vi "Connect to Error Handles.vi"(8 "error in":errorcluster, 9 "Timeout (ms)":u16, 11 "VS Plugin Inline Async API in":refnum<class "VS Plugin Inline Async API.lvclass">) -> (0 "error out":errorcluster, 3 "VS Plugin Inline Async API out":refnum<class "VS Plugin Inline Async API.lvclass">)   [LabVIEW 2024, in "VS Plugin Inline Async API.lvlib" / "VS Plugin Inline Async API.lvclass"]
uses:
  VS Plugin Inline Async API.lvclass
  VS Plugin Inline Async API.lvclass/VS Plugin Inline Async API.ctl
  <vilib>/ErrorRing/Error Ring.xnode
  VS Plugin Inline Async API.lvlib
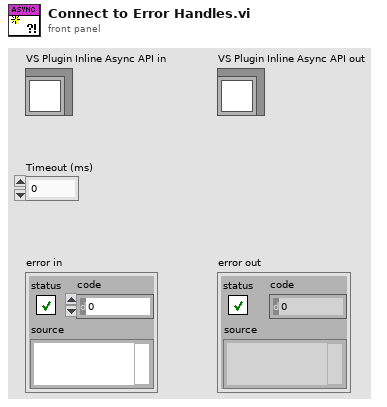
[diagram p1: front panel]
types:
  T1 = cluster{"read mode":enum16{"polling", "blocking"}, "write mode":enum16{"polling", "blocking"}}
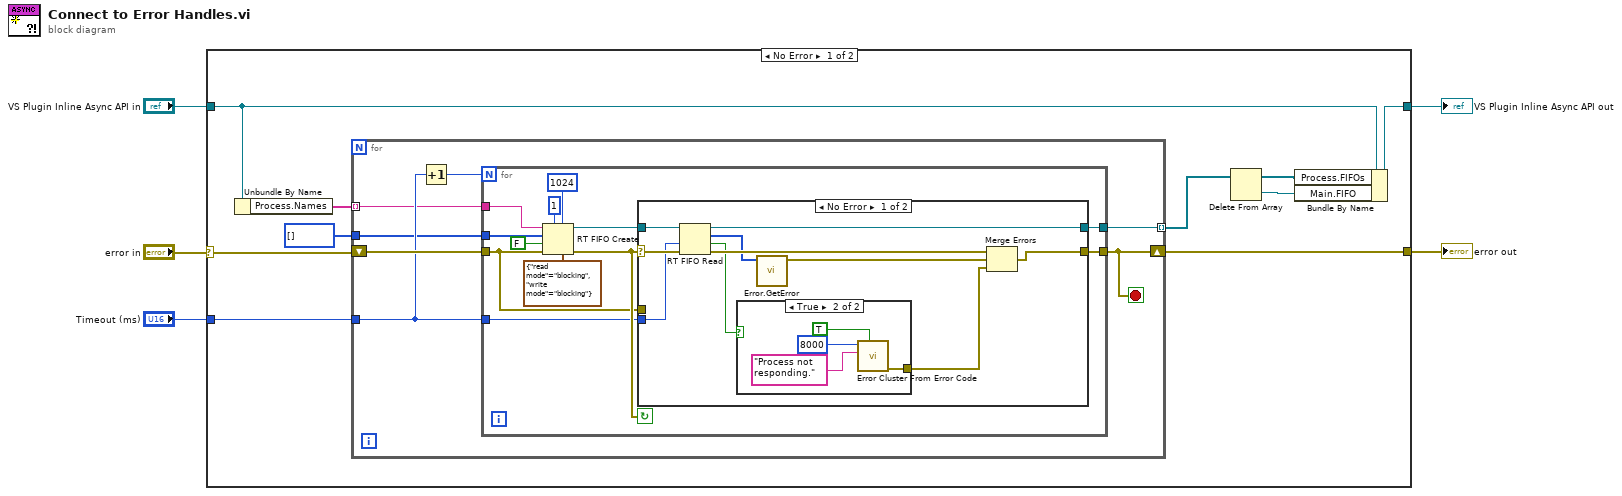
[diagram p0: block diagram]
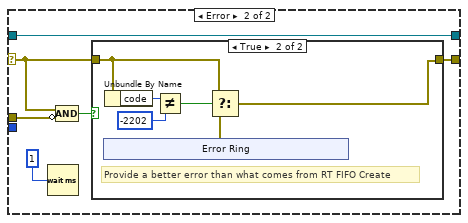
[diagram p3: hidden frame]
diagram:
  n1 = case shown="No Error" "error in" {
    selector: "error in" -> [w15 w67]
    tunnel: [w14 w67] -> w4
    tunnel: "Timeout (ms)" -> [w13 _]
    tunnel: "VS Plugin Inline Async API in" -> [w11 w66]
    tunnel: [w12 w66] -> w1
    frame No Error {
      n2 = Unbundle By Name(w11) -> ("Process.Names"=w10:string[])
      n3 = for {
        shift-right: [w21] -> w14
        shift-left: w15 -> [w22]
        tunnel: [w20] -> w9 mode=indexing
        tunnel: w13 -> [w18]
        tunnel: w10 -> [w17] mode=indexing
        tunnel: u8[] [] -> [w16]
        stop <- w21 stop-if-true
        n4 = Increment(x=w18) -> (x+1=w19:u16)
        n5 = for {
          N: w19 -> [_]
          tunnel: [w30] -> w20
          tunnel: w18 -> [w28]
          tunnel: w22 -> [w32]
          tunnel: [w34] -> w21
          tunnel: w17 -> [w27]
          tunnel: w16 -> [w24]
          stop <- w33 continue-if-true
          n6 = RT FIFO Create(0:w27, 1:w24, 2:FALSE ("create if not found? (T)"), 3:w32, 4:u32 1 ("size (10)"), 6:u32 1024 ("elements in array (1)"), 7:T1 {"read mode"=enum."blocking", "write mode"=enum."blocking"} ("r/w modes (polling,polling)")) -> (8:w29:refnum<k33>, 11:w33:errorcluster)  [unwired: 1 in, 1 out]
          n7 = case shown="No Error" w33 {
            selector: w33 -> [w44 w53]
            tunnel: [w42 w52] -> w34
            tunnel: [w38 w51] -> w30
            tunnel: w29 -> [w39 w51]
            tunnel: w28 -> [w37 _]
            tunnel: w32 -> [_ w54]
            frame No Error {
              n8 = RT FIFO Read(0:w39, 2:w37, 3:w44) -> (8:w38:refnum<k33>, 9:w35:u8[], 10:w36:bool, 11:w43:errorcluster)  [unwired: 1 in, 1 out]
              n9 = case shown="True" w36 {
                tunnel: [_ w48] -> w41
                frame False {
                }
                frame True {
                  n10 = call <vilib>:"Error Cluster From Error Code.vi"("show call chain? (False)"=TRUE, "error message (\"\")"="Process not responding." ("source"), "error code (0)"=8000) -> ("error out"=w48:errorcluster)  [unwired: 6 in]
                }
              }
              n11 = call "Error.GetError.vi"("Msg"=w35) -> ("error out"=w40:errorcluster)  [unwired: 10 in]
              n12 = Merge Errors(w43, w40, w41) -> (w42:errorcluster)
            }
            frame Error {
              n13 = Wait (ms)(milliseconds to wait=u32 1) -> ()  [unwired: 1 out]
              n14 = Compound Arithmetic op=AND(w53, invert w54) -> (w49:bool)
              n15 = case shown="True" w49 {
                tunnel: w53 -> [w55 w61]
                tunnel: [w55 w59] -> w52
                frame False {
                  # "No new error from RT FIFO Create"
                }
                frame True {
                  # "Provide a better error than what comes from RT FIFO Create"
                  n16 = xnode "Error Ring"() -> ("error out"=w60:errorcluster)
                  n17 = Unbundle By Name(w61) -> ("code"=w58:i32)
                  n18 = Not Equal?(x=w58, y=-2202) -> (x != y?=w56:bool)
                  n19 = Select(t=w61, s=w56, f=w60) -> (s? t:f=w59:errorcluster)
                }
              }
            }
          }
        }
      }
      n20 = Delete From Array(array=w9) -> (deleted portion=w8:refnum<k33>, array with subset deleted=w7:refnum<k33>[])  [unwired: 2 in]
      n21 = Bundle By Name(cluster=w11, "Process.FIFOs"=w7, "Main.FIFO"=w8) -> (w12:refnum<class "VS Plugin Inline Async API.lvclass">)
    }
    frame Error {
    }
  }
  "error out" <- w4
  "VS Plugin Inline Async API out" <- w1
